vi "SimpleGraphFacade.vi"(0 "Data In":T4 {"Settings"."Time" format="%<%H:%M\n%d/%m/%y>T"}, 2 "Display State In":T2, 3 "Container State":T3) -> (6 "Data Out":T4 {"Settings"."Time" format="%<%H:%M\n%d/%m/%y>T"}, 7 "Display State Out":T2, 8 "Action":T1)   [LabVIEW 2014, in "SimpleView.xctl"]
uses:
  <userlib>/CurtinCode/SimpleViewctrl/SimpleView.xctl
  <userlib>/CurtinCode/SimpleViewctrl/SimpleGraphData.ctl
  <userlib>/CurtinCode/DataControl.ctl
  <userlib>/CurtinCode/SettingsControl.ctl
  <vilib>/_xctls/Container State.ctl
  <userlib>/CurtinCode/SimpleViewctrl/SimpleGraphState.ctl
  <vilib>/_xctls/Action.ctl
  <vilib>/_xctls/XControlSupport.lvlib
panel:
  out "Magnitude":cluster{i32, dbl, "data":dbl[]}[](graph)
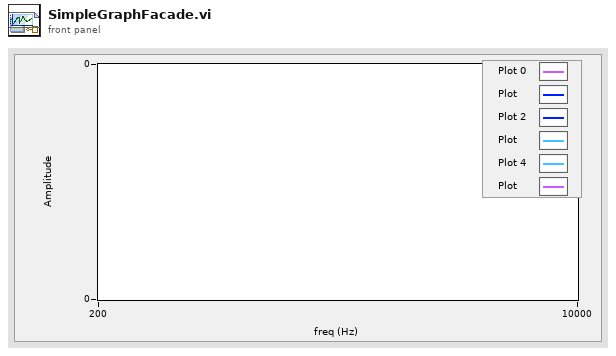
[diagram p1: front panel]
types:
  T1 = typedef "XControlSupport.lvlib/Action.ctl" = cluster{"Data Changed?":bool, "State Changed?":bool, "Action Name":string}
  T2 = typedef "SimpleView.xctl/SimpleGraphState.ctl" = cluster{"Numeric":dbl}
  T3 = typedef "XControlSupport.lvlib/Container State.ctl" = cluster{"Indicator?":bool, "Run Mode?":bool, " Refnum":refnum<vi>}
  T4 = typedef "SimpleView.xctl/SimpleGraphData.ctl" = T5[]
  T5 = typedef "DataControl.ctl" = cluster{"Settings":T6, "Data":cluster{i32, dbl, "data":dbl[]}[], "Plot type":enum16{"Linear", "log"}}
  T6 = typedef "SettingsControl.ctl" = cluster{"Data Path":path, "Time":timestamp, "Sampling Rate (Hz)":u16, "Device":u16, "pre-trigger (sec)":dbl, "length of sample (sec)":dbl, "trigger value (V)":dbl, "Labels":string[], "Cutoffs (sec)":dbl[], "Freq Bands":dbl[]}
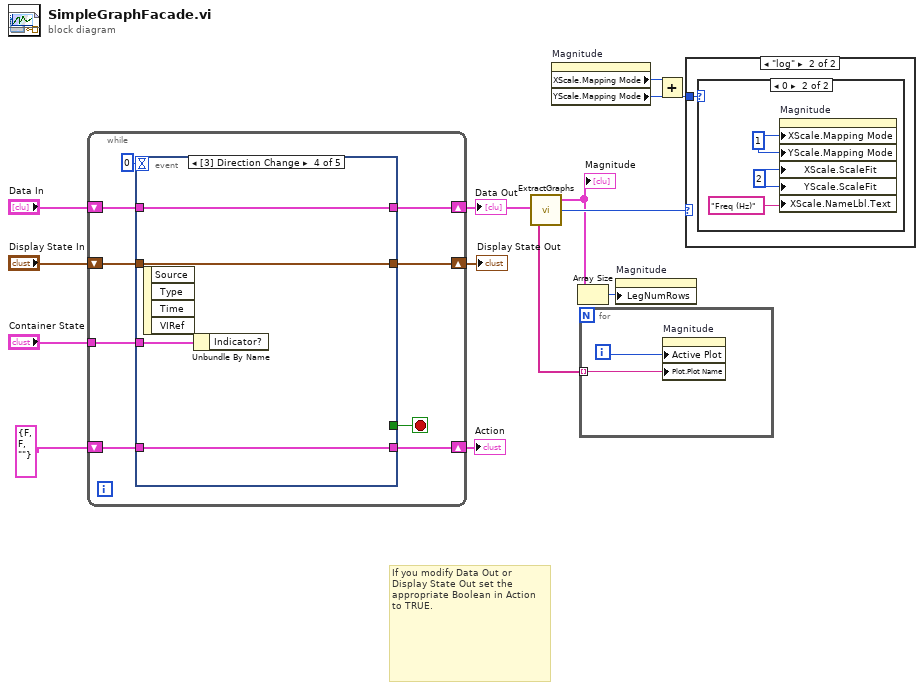
[diagram p0: block diagram]
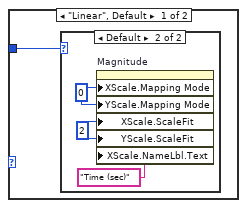
[diagram p2: hidden frame]
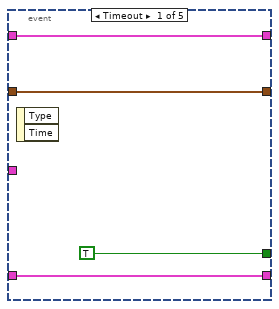
[diagram p5: hidden frame]
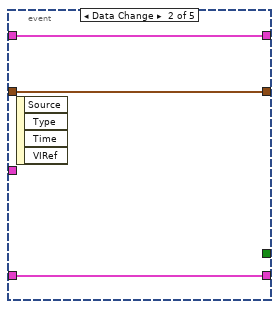
[diagram p6: hidden frame]
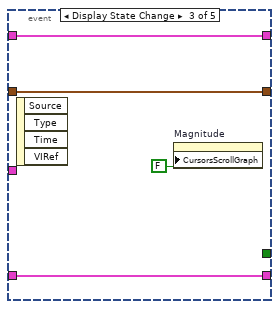
[diagram p7: hidden frame]
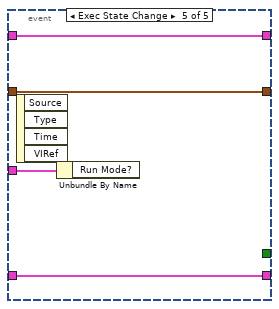
[diagram p8: hidden frame]
diagram:
  # "If you modify Data Out or\nDisplay State Out set the\nappropriate Boolean in Action\nto TRUE."
  n1 = while {
    shift-right: [w22] -> w12
    shift-left: "Display State In" -> [w23]
    tunnel: "Container State" -> [w19]
    shift-right: [w17] -> w8
    shift-left: "Data In" -> [w18]
    shift-right: [w15] -> w10
    shift-left: T1 {"Data Changed?"=FALSE, "State Changed?"=FALSE, "Action Name"=""} ("Action") -> [w16]
    stop <- w21 stop-if-true
    n2 = event shown="[3] Direction Change" {
      selector: _ -> [_ _ _ _ _]
      dyn-events: _ -> [_ _ _ _ _]
      timeout: 0 -> [_ _ _ _ _]
      tunnel: w23 -> [w25 w29 w34 w37 w41]
      tunnel: [w25 w29 w34 w37 w41] -> w22
      tunnel: [TRUE _ _ _ _] -> w21
      tunnel: w19 -> [_ _ _ w38 w42]
      tunnel: w18 -> [w24 w30 w33 w36 w40]
      tunnel: [w24 w30 w33 w36 w40] -> w17
      tunnel: [w26 w28 w32 w35 w39] -> w15
      tunnel: w16 -> [w26 w28 w32 w35 w39]
      event Timeout {
        n3 = event-data() -> ()  [unwired: 1 in, 2 out]
      }
      event Data Change {
        n4 = event-data() -> ()  [unwired: 1 in, 4 out]
      }
      event Display State Change {
        n5 = event-data() -> ()  [unwired: 1 in, 4 out]
        n6 = property on="Magnitude" class="WFGraph (strict)"("CursorsScrollGraph"=FALSE ("Cursors Scroll Graph")) -> ()  [unwired: 2 in, 2 out]
      }
      event Direction Change {
        n7 = event-data() -> ()  [unwired: 1 in, 4 out]
        n8 = Unbundle By Name(w38) -> ()  [unwired: 1 out]
      }
      event Exec State Change {
        n9 = event-data() -> ()  [unwired: 1 in, 4 out]
        n10 = Unbundle By Name(w42) -> ()  [unwired: 1 out]
      }
    }
  }
  "Display State Out" <- w12
  "Action" <- w10
  "Data Out" <- w8
  n11 = call <userlib>:"ExtractGraphs.vi"("Spectra Out"=w8) -> ("Plot Labels"=w1:string[], "Mag"=w3:cluster{i32, dbl, "data":dbl[]}[], "Plot type"=w7:enum16{"Linear", "log"})  [unwired: 1 out]
  "Magnitude" <- w3
  n12 = property on="Magnitude" class="WFGraph (strict)"() -> ("XScale.Mapping Mode"=w6:u8, "YScale.Mapping Mode"=w5:u8)  [unwired: 2 in, 2 out]
  n13 = Array Size(array=w3) -> (size(s)=w2:i32)
  n14 = for {
    tunnel: w1 -> [w44] mode=indexing
    i -> [w43]
    n15 = property on="Magnitude" class="WFGraph (strict)"("Active Plot"=w43, "Plot.Plot Name"=w44) -> ()  [unwired: 2 in, 2 out]
  }
  n16 = property on="Magnitude" class="WFGraph (strict)"("LegNumRows"=w2) -> ()  [unwired: 2 in, 2 out]
  n17 = Add(x=w6, y=w5) -> (x+y=w4:u8)
  n18 = case shown="\"log\"" w7 {
    tunnel: w4 -> [w45 w49]
    frame "Linear", Default {
      n19 = case shown="Default" w45 {
        frame 0 {
        }
        frame Default {
          w47 = u8 2 ("X Scale.Mapping Mode")
          w48 = u8 0 ("X Scale.Mapping Mode")
          n20 = property on="Magnitude" class="WFGraph (strict)"("XScale.Mapping Mode"=w48, "YScale.Mapping Mode"=w48, "XScale.ScaleFit"=w47, "YScale.ScaleFit"=w47, "XScale.NameLbl.Text"="Time (sec)" ("X Scale.Unit Label.Text")) -> ()  [unwired: 2 in, 2 out]
        }
      }
    }
    frame "log" {
      n21 = case shown="0" w49 {
        frame Default {
        }
        frame 0 {
          w51 = u8 2 ("X Scale.Mapping Mode")
          w52 = u8 1 ("X Scale.Mapping Mode")
          n22 = property on="Magnitude" class="WFGraph (strict)"("XScale.Mapping Mode"=w52, "YScale.Mapping Mode"=w52, "XScale.ScaleFit"=w51, "YScale.ScaleFit"=w51, "XScale.NameLbl.Text"="Freq (Hz)" ("X Scale.Unit Label.Text")) -> ()  [unwired: 2 in, 2 out]
        }
      }
    }
  }
